vi "Instantiate RTV.vi"(0 "RT Variables in":refnum<class "RT Variables.lvclass">, 11 "error in (no error)":errorcluster) -> (4 "RT Variables out":refnum<class "RT Variables.lvclass">, 15 "error out":errorcluster)   [LabVIEW 2019, in "LSL.lvlib" / "RT Variables.lvclass"]
uses:
  RT Variables.lvclass
  RT Variables.lvclass/RT Variables.ctl
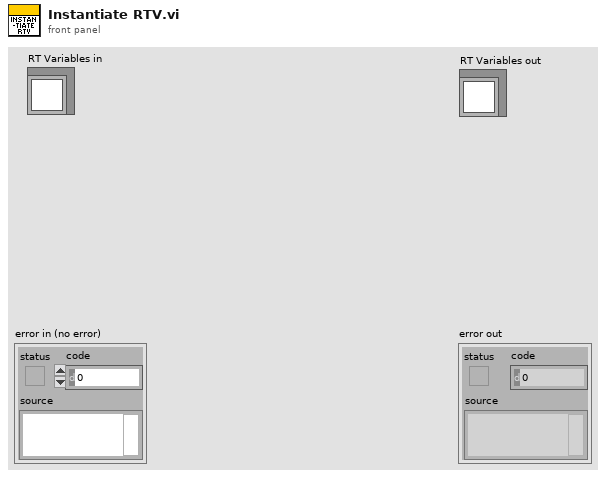
[diagram p1: front panel]
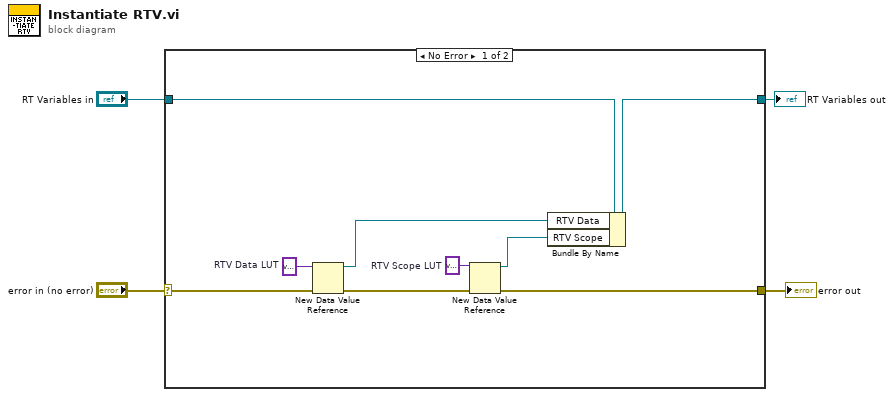
[diagram p0: block diagram]
diagram:
  n1 = case shown="No Error" "error in (no error)" {
    selector: "error in (no error)" -> [w6 w15]
    tunnel: [w11 w15] -> w3
    tunnel: "RT Variables in" -> [w8 w14]
    tunnel: [w7 w14] -> w1
    frame No Error {
      w12 = variant  # RTV Scope LUT
      w13 = variant  # RTV Data LUT
      n2 = New Data Value Reference(data value=w13, error in=w6) -> (data value reference=w10:refnum<data-value>, error out=w5:errorcluster)
      n3 = New Data Value Reference(data value=w12, error in=w5) -> (data value reference=w9:refnum<data-value>, error out=w11:errorcluster)
      n4 = Bundle By Name(cluster=w8, "RTV Data"=w10, "RTV Scope"=w9) -> (w7:refnum<class "RT Variables.lvclass">)
    }
    frame Error {
    }
  }
  "error out" <- w3
  "RT Variables out" <- w1
